vi "Config Transductores.vi"(11 "Transductores":bool[][](array[boolean]) caption="TRANSDUCTORES") -> (3 "Transductores Out":bool[][](array[boolean]) caption="TRANSDUCTORES")   [LabVIEW 2014, in "CAP-USB-1.lvlib" / "CAP-USB-1.lvclass"]
doc: "Pantalla de configuracion de Transductores"
uses:
  CAP-USB-1Class/CAP-USB-1.lvclass
panel:
  in  "Cancelar":bool
  in  "Config Transductores":bool
  # "1-16"
  # "17-32"
  # "33-48"
  # "49-64"
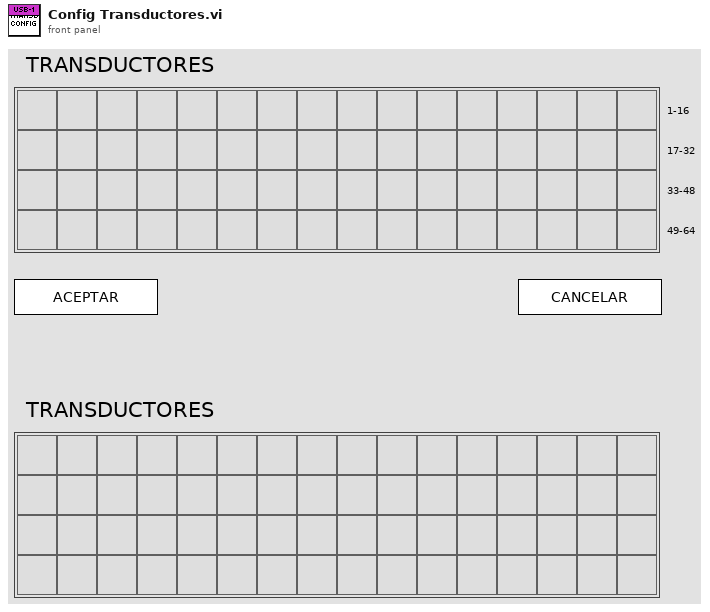
[diagram p1: front panel]
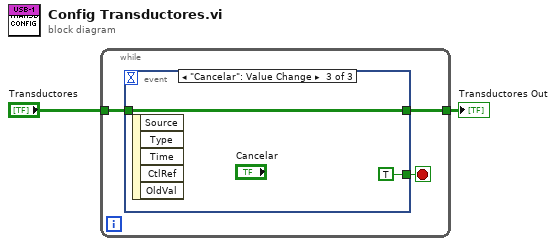
[diagram p0: block diagram]
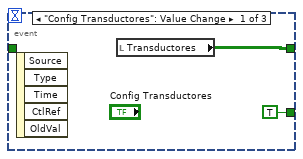
[diagram p2: hidden frame]
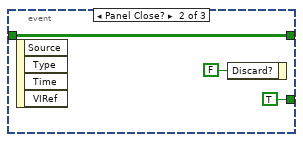
[diagram p3: hidden frame]
diagram:
  n1 = while {
    tunnel: [w4] -> w2
    tunnel: "Transductores" -> [w3]
    stop <- w5 stop-if-true
    n2 = event shown="[2] \"Cancelar\": Value Change" {
      selector: _ -> [_ _ _]
      dyn-events: _ -> [_ _ _]
      timeout: _ -> [_ _ _]
      tunnel: [TRUE ("Config Transductores") TRUE ("Config Transductores") TRUE ("Config Transductores")] -> w5
      tunnel: [w7 w8 w11] -> w4
      tunnel: w3 -> [_ w8 w11]
      event "Config Transductores": Value Change {
        n3 = event-data() -> ()  [unwired: 1 in, 5 out]
        n4 = local read "Transductores"() -> (w7:bool[][])
      }
      event Panel Close? {
        n5 = event-data() -> ()  [unwired: 1 in, 4 out]
        n6 = event-data("Discard?"=FALSE) -> ()  [unwired: 1 in, 1 out]
      }
      event "Cancelar": Value Change {
        n7 = event-data() -> ()  [unwired: 1 in, 5 out]
      }
    }
  }
  "Transductores Out" <- w2
